vi "DIGITIZER_READ.vi"(2 "min record length":i32, 3 "trigger type":enum16{"Edge", "Digital", "Immediate"}(ring), 4 "error in":errorcluster, 5 "DIG CHANNELS":string, 6 "DIG USED?":bool, 7 "DIG REF":refnum<k15>) -> (0 "error out":errorcluster, 1 "waveform":T1(array[cluster]))   [LabVIEW 2010]
uses:
  <instrlib>/niScope/Acquire/niScope Multi Read Cluster.vi
  <instrlib>/niScope/Acquire/Fetch/niScope Multi Fetch Cluster.vi
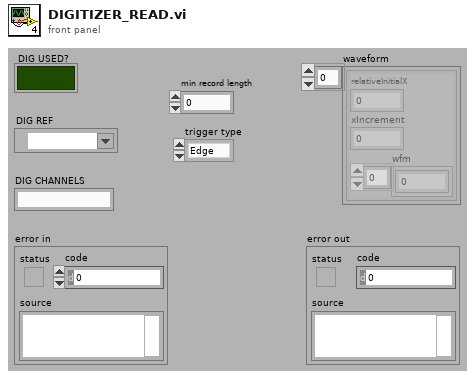
[diagram p1: front panel]
types:
  T1 = cluster{"relativeInitialX":dbl, "xIncrement":dbl, "wfm":dbl[]}[]
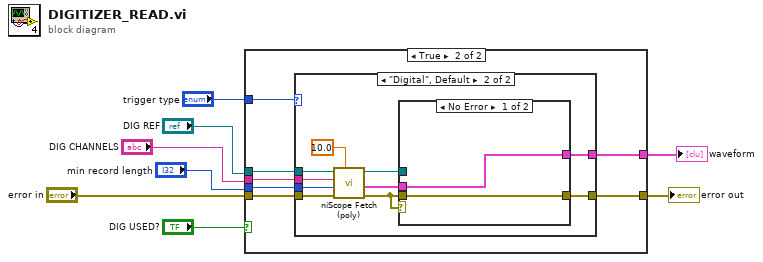
[diagram p0: block diagram]
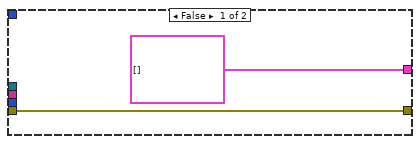
[diagram p2: hidden frame]
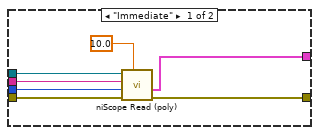
[diagram p3: hidden frame]
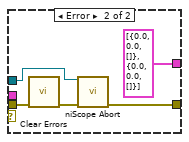
[diagram p4: hidden frame]
diagram:
  n1 = case shown="True" "DIG USED?" {
    tunnel: "DIG CHANNELS" -> [_ w16]
    tunnel: "error in" -> [w10 w14]
    tunnel: "DIG REF" -> [_ w17]
    tunnel: [w10 w12] -> w2
    tunnel: [T1 [] ("waveform") w13] -> w1
    tunnel: "min record length" -> [_ w15]
    tunnel: "trigger type" -> [_ w11]
    frame False {
    }
    frame True {
      n2 = case shown="\"Digital\", Default" w11 {
        tunnel: w17 -> [w24 w34]
        tunnel: w16 -> [w23 w33]
        tunnel: w15 -> [w22 w32]
        tunnel: w14 -> [w21 w31]
        tunnel: [w19 w26] -> w13
        tunnel: [w18 w29] -> w12
        frame "Immediate" {
          n3 = call-poly <instrlib>:"niScope Read (poly).vi"("timeout"=10.0, "error in"=w21, "numSamples"=w22, "channels"=w23, "instrument handle"=w24) -> ("error out"=w18:errorcluster, "waveform"=w19:T1)  [unwired: 3 in, 2 out]
        }
        frame "Digital", Default {
          n4 = call-poly <instrlib>:"niScope Fetch (poly).vi"("timeout"=10.0, "error in"=w31, "numSamples"=w32, "channels"=w33, "instrument handle"=w34) -> ("error out"=w28:errorcluster, "waveform"=w27:T1, "instrument handle out"=w25:refnum<k15>)  [unwired: 3 in, 1 out]
          n5 = case shown="No Error" w28 {
            tunnel: w28 -> [w35 w41]
            tunnel: [w35 w38] -> w29
            tunnel: w27 -> [w36 _]
            tunnel: [w36 T1 [{"relativeInitialX"=0.0, "xIncrement"=0.0, "wfm"=[]}, {"relativeInitialX"=0.0, "xIncrement"=0.0, "wfm"=[]}] ("waveform")] -> w26
            tunnel: w25 -> [_ w37]
            frame No Error {
            }
            frame Error {
              n6 = call <vilib>:"Clear Errors.vi"("error in (no error)"=w41) -> ("error out"=w39:errorcluster)  [unwired: 6 in]
              n7 = call <instrlib>:"niScope Abort.vi"("instrument handle"=w37, "error in"=w39) -> ("error out"=w38:errorcluster)  [unwired: 12 in, 1 out]
            }
          }
        }
      }
    }
  }
  "error out" <- w2
  "waveform" <- w1
